vi "isDeviceActive.vi"(8 "error in (no error)":errorcluster, 11 "device in":refnum<class "device.lvclass">) -> (0 "error out":errorcluster, 2 "active":bool, 3 "device out":refnum<class "device.lvclass">)   [LabVIEW 2009, in "Tools.lvlib" / "DatabaseHelpers.lvlib" / "device.lvclass"]
uses:
  device.lvclass
  Scripting/ScriptingEvent/ScriptEventList/ScriptEventList.lvclass
  device.lvclass/device.ctl
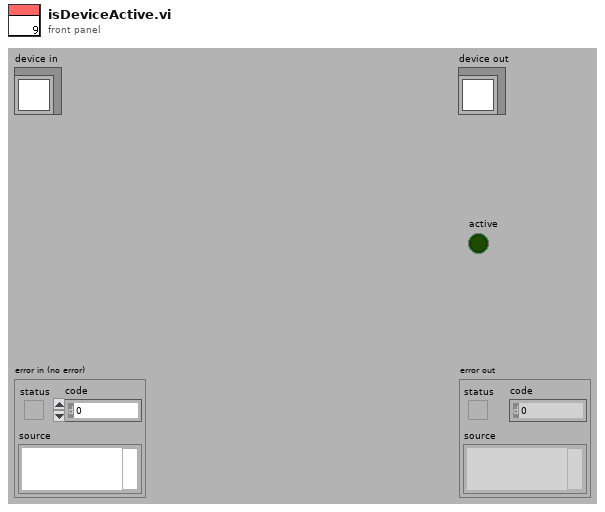
[diagram p1: front panel]
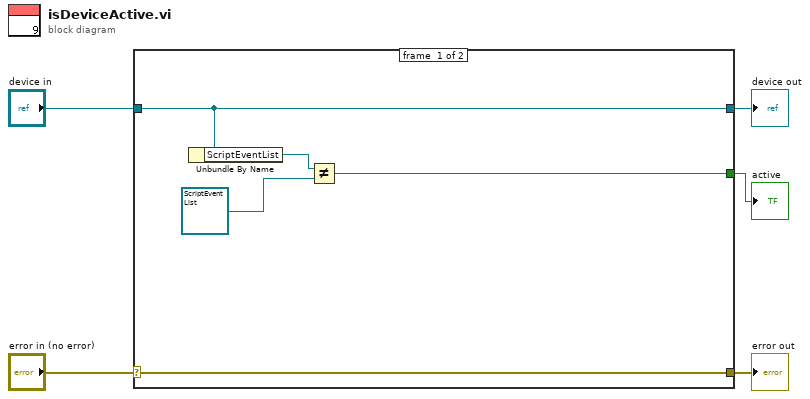
[diagram p0: block diagram]
diagram:
  n1 = case shown="No Error" "error in (no error)" {
    selector: "error in (no error)" -> [w10 w12]
    tunnel: [w10 w12] -> w4
    tunnel: [w9 w11] -> w2
    tunnel: "device in" -> [w9 w11]
    tunnel: [w6 _] -> w1
    frame #0 {
      n2 = Unbundle By Name(w9) -> ("ScriptEventList"=w8:refnum<class "ScriptEventList.lvclass">)
      n3 = Not Equal?(x=w8, y=refnum<class "ScriptEventList.lvclass"> refnum ("Tools.lvlib:Scripting.lvlib:ScriptEventList.lvclass")) -> (x != y?=w6:bool)
    }
    frame #1 {
    }
  }
  "error out" <- w4
  "device out" <- w2
  "active" <- w1
